vi "Update Test Name if Not Defined.vi"(8 "error in":errorcluster, 10 "Caller (Non-VIM)":T1=1 items=["Non VIM  Caller"=1, "VIM Caller"=0], 11 "Options in":refnum<class "Options.lvclass">) -> (0 "error out":errorcluster, 3 "Options out":refnum<class "Options.lvclass">)   [LabVIEW 2020, in "Approval Tests.lvlib" / "Options.lvclass"]
uses:
  Options.lvclass
  Options.lvclass/Options.ctl
  Naming Data/Naming Data.lvclass
  Caller.ctl
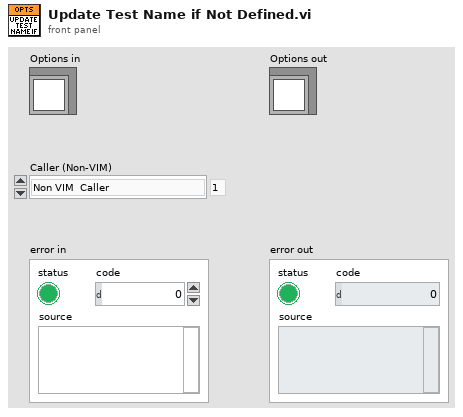
[diagram p1: front panel]
types:
  T1 = typedef "Approval Tests.lvlib/Options.lvclass/Caller.ctl" = u16
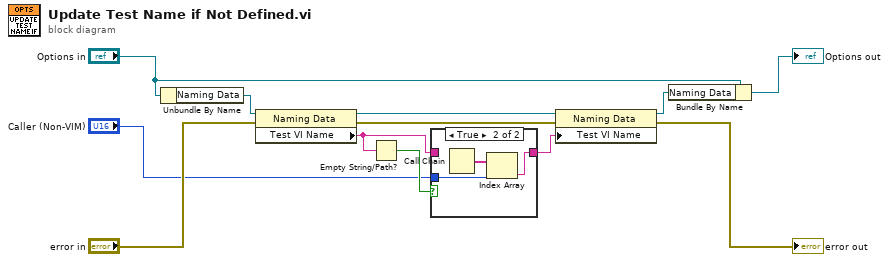
[diagram p0: block diagram]
diagram:
  n1 = Unbundle By Name("Options in") -> ("Naming Data"=w5:refnum<class "Naming Data.lvclass">)
  n2 = property class="Naming Data"(reference=w5, error in="error in") -> (reference out=w3:refnum<class "Naming Data.lvclass">, error out=w11:errorcluster, "Test VI Name"=w4:string)
  n3 = Empty String/Path?(string/path=w4) -> (empty?=w8:bool)
  n4 = case shown="True" w8 {
    tunnel: w4 -> [w13 _]
    tunnel: [w13 w16] -> w2
    tunnel: "Caller (Non-VIM)" -> [_ w14]
    frame False {
    }
    frame True {
      n5 = Call Chain() -> (call chain=w15:string[])
      n6 = Index Array(array=w15, index=w14) -> (element=w16:string)
    }
  }
  n7 = property class="Naming Data"(reference=w3, error in=w11, "Test VI Name"=w2) -> (reference out=w1:refnum<class "Naming Data.lvclass">, error out=→"error out":errorcluster)
  n8 = Bundle By Name(cluster="Options in", "Naming Data"=w1) -> (→"Options out":refnum<class "Options.lvclass">)
